vi "Purge and Defragment.vi"(8 "error in":errorcluster, 10 "Path":path, 11 "TDMS in":refnum<class "TDMS.lvclass">) -> (0 "error out":errorcluster, 3 "TDMS out":refnum<class "TDMS.lvclass">)   [LabVIEW 2019, in "TDMS.lvlib" / "TDMS.lvclass"]
uses:
  TDMS.lvclass
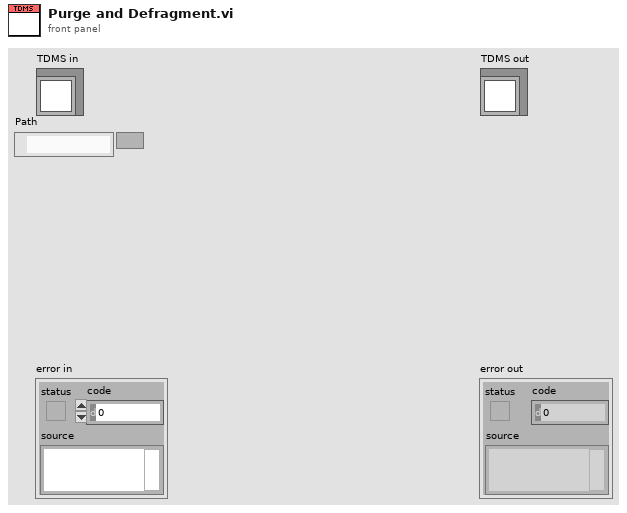
[diagram p1: front panel]
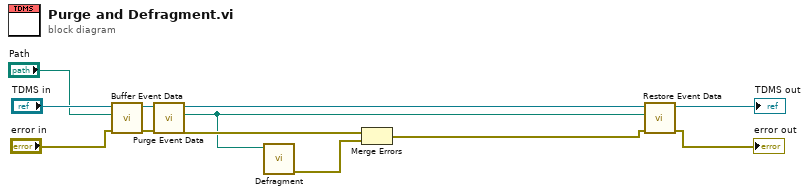
[diagram p0: block diagram]
diagram:
  n1 = call "Buffer Event Data.vi"("error in"="error in", "Path"="Path", "TDMS in"="TDMS in") -> ("error out"=w11:errorcluster, "TDMS out"=w12:refnum<class "TDMS.lvclass">)  [unwired: 7 in]
  n2 = call "Purge Event Data.vi"("error in"=w11, "TDMS in"=w12) -> ("error out"=w5:errorcluster, "file path out"=w3:path, "TDMS out"=w9:refnum<class "TDMS.lvclass">)  [unwired: 7 in]
  n3 = call "Defragment.vi"("Path"=w3) -> ("error out"=w4:errorcluster)  [unwired: 10 in]
  n4 = Merge Errors(w5, w4) -> (w2:errorcluster)
  n5 = call "Restore Event Data.vi"("error in"=w2, "Path"=w3, "TDMS in"=w9) -> ("error out"=→"error out":errorcluster, "TDMS out"=→"TDMS out":refnum<class "TDMS.lvclass">)  [unwired: 7 in]
